vi "Queue Ball Element cam3.vi"(8 "error in (no error)":errorcluster, 11 "Image in":T1) -> (0 "error out":errorcluster)   [LabVIEW 2023]
uses:
  <vilib>/vision/Image Controls.llb/IMAQ Image.ctl
panel:
  out "queue out":refnum<queue>
  in  "queue":refnum<queue>
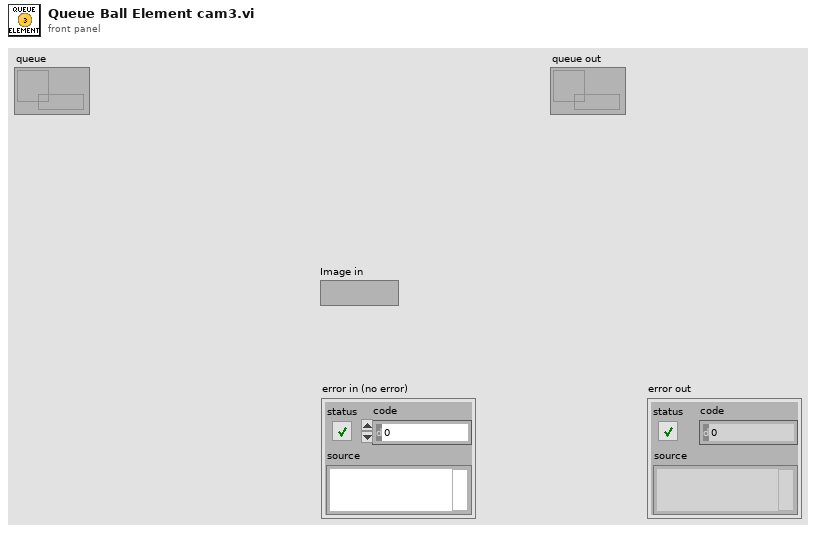
[diagram p1: front panel]
types:
  T1 = typedef "IMAQ Image.ctl" = refnum<image>
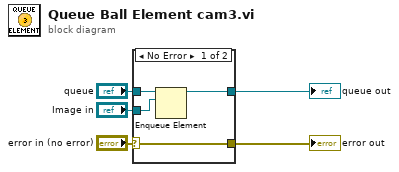
[diagram p0: block diagram]
diagram:
  n1 = case shown="No Error" "error in (no error)" {
    selector: "error in (no error)" -> [w9 w11]
    tunnel: [w9 w11] -> w4
    tunnel: "Image in" -> [w8 _]
    tunnel: "queue" -> [w7 w10]
    tunnel: [w6 w10] -> w1
    frame No Error {
      n2 = Enqueue Element(queue=w7, element=w8) -> (queue out=w6:refnum<queue>)  [unwired: 2 in, 2 out]
    }
    frame Error {
    }
  }
  "error out" <- w4
  "queue out" <- w1
